vi "Get Possible Targets.vi"(11 "Targets Used":T1[](array[typedef])) -> (3 "Possible Targets":T2(array[ring]))   [LabVIEW 2015, in "Configuration Tool.lvlib"]
uses:
  Configuration Tool.lvlib
  XML Controls/Supported Targets.ctl
  VeriStand XML Parser.lvlib
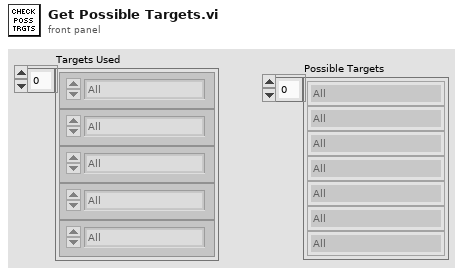
[diagram p1: front panel]
types:
  T1 = typedef "VeriStand XML Parser.lvlib/Supported Targets.ctl" = enum16{"All", "Pharlap", "VxWorks", "Windows", "Linux_32_ARM", "Linux_x64", "PharlapWindows", "PharlapVxWorks", "VxWorksWindows"}
  T2 = enum16{"All", "Pharlap", "VxWorks", "Windows", "Linux_32_ARM", "Linux_x64", "PharlapWindows", "PharlapVxWorks", "VxWorksWindows"}[]
  T3 = enum16{"All", "Pharlap", "VxWorks", "Windows", "Linux_32_ARM", "Linux_x64", "PharlapWindows", "PharlapVxWorks", "VxWorksWindows"}
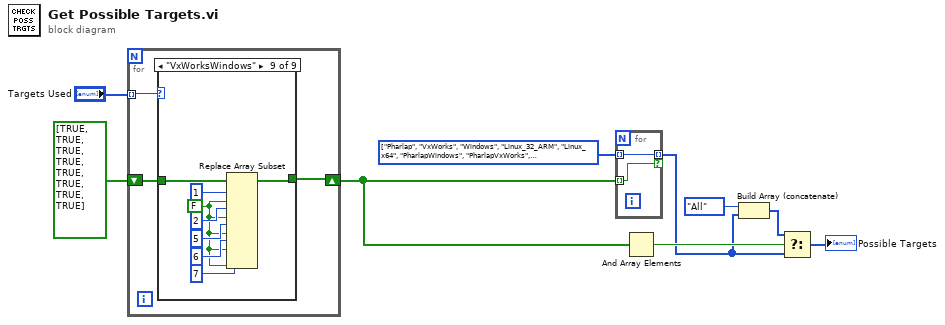
[diagram p0: block diagram]
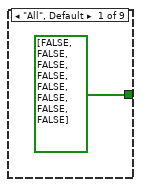
[diagram p2: hidden frame]
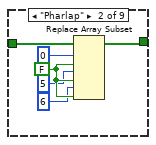
[diagram p3: hidden frame]
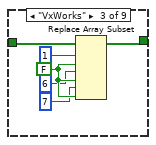
[diagram p4: hidden frame]
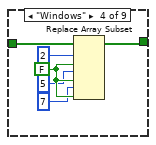
[diagram p5: hidden frame]
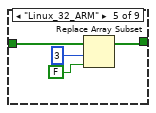
[diagram p6: hidden frame]
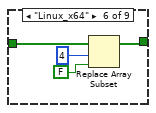
[diagram p7: hidden frame]
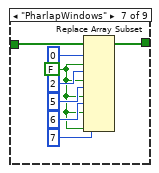
[diagram p8: hidden frame]
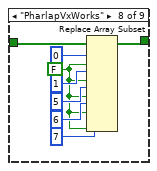
[diagram p9: hidden frame]
diagram:
  w8 = T2 [enum."Pharlap", enum."VxWorks", enum."Windows", enum."Linux_32_ARM", enum."Linux_x64", enum."PharlapWindows", enum."PharlapVxWorks", enum."VxWorksWindows"] items=["All", "Pharlap", "VxWorks", "Windows", "Linux_32_ARM", "Linux_x64", "PharlapWindows", "PharlapVxWorks", "VxWorksWindows"]
  n1 = for {
    shift-right: [w11] -> w7
    shift-left: bool[] [TRUE, TRUE, TRUE, TRUE, TRUE, TRUE, TRUE, TRUE] -> [w12]
    tunnel: "Targets Used" -> [w10] mode=indexing
    n2 = case shown="\"VxWorksWindows\"" w10 {
      tunnel: w12 -> [_ w19 w21 w26 w35 w37 w44 w51 w57]
      tunnel: [bool[] [FALSE, FALSE, FALSE, FALSE, FALSE, FALSE, FALSE, FALSE] w14 w20 w27 w34 w36 w43 w50 w56] -> w11
      frame "All", Default {
      }
      frame "Pharlap" {
        w17 = FALSE
        n3 = Replace Array Subset(array=w19, new element #1=w17, index #1=0 ("index"), new element #2=w17, index #2=5 ("index"), new element #3=w17, index #3=6 ("index")) -> (w14:bool[])
      }
      frame "VxWorks" {
        w24 = FALSE
        n4 = Replace Array Subset(array=w21, new element #1=w24, index #1=1 ("index"), new element #2=w24, index #2=6 ("index"), new element #3=w24, index #3=7 ("index")) -> (w20:bool[])
      }
      frame "Windows" {
        w30 = FALSE
        n5 = Replace Array Subset(array=w26, new element #1=w30, index #1=2 ("index"), new element #2=w30, index #2=5 ("index"), new element #3=w30, index #3=7 ("index")) -> (w27:bool[])
      }
      frame "Linux_32_ARM" {
        n6 = Replace Array Subset(array=w35, new element=FALSE, index=3) -> (w34:bool[])
      }
      frame "Linux_x64" {
        n7 = Replace Array Subset(array=w37, new element=FALSE, index=4) -> (w36:bool[])
      }
      frame "PharlapWindows" {
        w41 = FALSE
        n8 = Replace Array Subset(array=w44, new element #1=w41, index #1=0 ("index"), new element #2=w41, index #2=2 ("index"), new element #3=w41, index #3=5 ("index"), new element #4=w41, index #4=6 ("index"), new element #5=w41, index #5=7 ("index")) -> (w43:bool[])
      }
      frame "PharlapVxWorks" {
        w49 = FALSE
        n9 = Replace Array Subset(array=w51, new element #1=w49, index #1=0 ("index"), new element #2=w49, index #2=1 ("index"), new element #3=w49, index #3=5 ("index"), new element #4=w49, index #4=6 ("index"), new element #5=w49, index #5=7 ("index")) -> (w50:bool[])
      }
      frame "VxWorksWindows" {
        w59 = FALSE
        n10 = Replace Array Subset(array=w57, new element #1=w59, index #1=1 ("index"), new element #2=w59, index #2=2 ("index"), new element #3=w59, index #3=5 ("index"), new element #4=w59, index #4=6 ("index"), new element #5=w59, index #5=7 ("index")) -> (w56:bool[])
      }
    }
  }
  n11 = for {
    tunnel: w7 -> [w64] mode=indexing
    tunnel: w8 -> [w65] mode=indexing
    tunnel: [w65] -> w4 mode=indexing if=w64
  }
  n12 = And Array Elements(Boolean array=w7) -> (logical AND=w6:bool)
  n13 = Build Array (concatenate)(T3."All" ("Supported Target"), w4) -> (w3:T2)
  n14 = Select(t=w3, s=w6, f=w4) -> (s? t:f=→"Possible Targets":T2)
